vi "EditorEinfachCRIO-11-15.vi"() -> ()   [LabVIEW 2010]
panel:
  out "error out":errorcluster
  in  "MethodeLöschen":bool
  in  "Metavariablen":string[](array[string])
  in  "MethodeDuplizieren":bool
  out "Methoden":T1(array[cluster]) {"FPGAPID"."proportional gain (Kc)" format="%.11g"; "FPGAPID"."integral gain (Kc*Ts/Ti)" format="%.11g"; "FPGAPID"."derivative gain (Kc*Td/Ts)" format="%.11g"}
  in  "T_MainMach2":dbl[](array[numeric])
  in  "t_MainMach2":dbl[](array[numeric])
  in  "T_MainMach1":dbl[](array[numeric])
  in  "t_MainMach1":dbl[](array[numeric])
  in  "EinstellungenSpeichern":bool
  out "LangsameHeizungen":string[](array[string])
  in  "AllesSpeichern":bool
  in  "ModuleLH":i32[](array[numeric]) min=1 max=3 step=1
  in  "NamenLangsameHeizungen":string[](array[string])
  out "Schnelle Heizungen":string[](array[string])
  in  "Modul3/AIsNamen":string[](array[string])
  in  "Modul2/AIsNamen":string[](array[string])
  in  "Modul1/AIsNamen":string[](array[string])
  in  "Methodenname":string
  in  "Int.Stop2":dbl
  in  "Int.Start2":dbl
  in  "Int.Stop1":dbl
  in  "Int.Start1":dbl
  in  "ZeitpktMS-2":dbl
  in  "ZeitpktMS-1":dbl
  in  "SPMPV":i32[](array[numeric])
  in  "ZeitpunkteMPV":dbl[](array[numeric])
  in  "Regler für den Probenfluß":i32
  in  "DateinameECD2":string
  in  "DateiordnerECD2":path
  in  "DateinameECD1":string
  in  "DateiordnerECD1":path
  in  "Wert2":dbl
  in  "Vergleichsoperator2":dbl(ring) items=["<", "<=", "=", ">=", ">", "=/="]
  in  "AbfragbareVariablen2":dbl(ring) items=["T1-Trap1", "T1-Trap2", "T1-StirlingKühlkopf", "T1-PreCol1", "T1-PreCol2", "T1-MainCol1a", "T1-MainCol1b", "T1-MainCol2a", "T1-MainCol2b", "T1-Bronkhorst1a", "T1-Bronkhorst1b", "T1-Bronkhorst2a", "T1-Bronkhorst2b", "T1-2Pos1B", "T1-Spare9", "T1-2Pos1A", "T1-Spare10", "T1-TurboPump", "T1-StirlingPlatine", "T1-Spare5", "T1-Spare6", "T1-Spare7", "T1-Spare8", "F1-MFM1", "F1-MFM0D [mL]", "P1-MethaneHP", "P1-MethaneLP", "P1-Vacuum", "TurboSpeed", "I1-MS-AC", "I1-Trap1", "I1-Trap2", "T2-ECD1a", "T2-ECD1b", "T2-ECD2a", "T2-ECD2b", "T2-Col1a", "T2-Col1b", "T2-Col2a", "T2-Col2b", "T2-Spare1", "T2-Spare2", "T2-Oven_a", "T2-Oven_b", "T2-Spare3", "T2-Spare4", "T2-Spare5", "F2-MFM0", "F2-MFM2A", "F2-MFM2B", "P2-N2O_HP", "P2-N2O_LP", "P2-CO2_HP", "P2-CO2_LP", "AI-Spare1", "FL-MFM1000mL", "AI-Spare3", "AI-Spare4", "StirlingAlarm", "StirlingEmerg.", "AI-Spare7", "AI-Spare8", "AI-Spare9", "FL-MFM30mL", "T0-DC/DC5", "I0-24V_M0", "I0-48V_M1", "I0-24V_M1", "I0-28V_M2", "T0-Spare3", "T0-Spare2", "T0-Spare4", "T0-DC/DC7", "I0-20V_Laptop", "I0-28V_M1", "I0-24V_M2", "I0-12V_Licor", "T0-Spare1", "T0-Drier", "T0-Spare5", "F0-MFM0A [L]", "TL-Licor_a", "P0-Span-HP", "P0-spare1", "P0-Stickstoff-LP", "P0-Helium-LP", "P0-Cal-HP", "P0-P9Tavco[bar]", "F0-MFM0B [L]", "TL-Licor_b", "P0-Span-LP", "P0-spare2", "P0-Stickstoff-HP", "P0-Helium-HP", "P0-Cal-LP", "F0-MFM3", "T-Trap1", "T-Trap2", "T-PreMach1", "T-PreMach2", "T-MainMach1", "T-MainMach2", "PrC0", "PrC0-Licor", "PrC1-Säule2", "PrC1-Säule1", "MFC1-Sample", "MFC1-Methan", "PrC1-BackFlush1", "PrC1-BackFlush2", "MFC2A", "MFC2B", "MFC2C", "PrC2A", "MFC2D", "MFC2E", "PrC2B", "Gesamte Zeit", "Methodenzeit", "Zykluszeit Mod0", "Zykluszeit Mod1", "Zykluszeit Mod2A", "Zykluszeit Mod2B", "PositionMPV", "OverflowB", "OverflowA", "StirlingAlarmAlarm!"]
  in  "Dateiname Housekeeping":string
  in  "Dateiordner Housekeeping":path=path "C:/Users/Atmos/Desktop/Johnny"
  in  "Startmethode":i32=1
  in  "Dateien fürs MS schicken?":bool
  in  "Zwangsbedingungen":dbl[][](array[numeric])
  out "ZwangsBedingungen":string[][](array[string])
  in  "löschen":bool
  in  "Bedingung Nr. X":i32
  in  "Bedingung übernehmen":bool
  in  "Ausgangswert":dbl
  in  "BedienbareVariablen":dbl(ring) items=["D0-48V_M1", "D0-28V_M1", "D0-Pump2", "DL-LiCalS1H", "D-Spare2", "D-Spare4", "D0-28V_M2", "D0-Pump1", "D0-S01/EV1", "DL-Licor", "D0-EV3", "D0-EV2", "D1-StopMS", "D1-StartMS", "D1-TrapEvac1", "D1-TrapEvac2", "D1-2Pos1A", "D1-2Pos1B", "D1-TurboPump", "D1-PrePump", "D1-VacPump1", "D1-VacPump2", "D1-Stirling", "D1-P_MS", "D1-S1B(7)", "D1-S1A(6)", "D1-S1G", "D1-Fan3", "D1-LüfterMach1", "D1-LüfterMach2", "D1-MS-Power", "D2-SpülflußA", "D2-2Pos2B", "D2-2Pos2A", "D2-ECD1HeaterOff", "D2-Fan1", "D2-Fan2", "D2-Probe2A", "D2-Probe2B", "D2-SpülflußB", "D2-ECD2HeaterOff", "Servo1 an", "Servo2 an", "Servo1 kalt", "Servo2 kalt", "Heizen?Trap1", "Heizen?Trap2", "Heizen?PreMach1", "Heizen?PreMach2", "Heizen?MainMach1", "Heizen?MainMach2", "Methodennummer", "STOPP!!!", "H1-Valve1B heizen?", "H1-Bronkhorst1 heizen?", "H1-Bronkhorst2 heizen?", "H1-Valve1A heizen?", "H0-Drier heizen?", "HL-Licor heizen?", "H2-ECD2 heizen?", "H2-Oven heizen?", "H2-Spare1 heizen?", "H2-Col2 heizen?", "H2-Col1 heizen?", "H2-ECD1 heizen?", "PrC0", "PrC0-Licor", "PrC1-Säule2", "PrC1-Säule1", "MFC1-Sample", "MFC1-Methan", "PrC1-BackFlush1", "PrC1-BackFlush2", "MFC2A", "MFC2B", "MFC2C", "PrC2A", "MFC2D", "MFC2E", "PrC2B", "PositionMPV", "OverflowB", "OverflowA", "StirlingAlarmAlarm!"]
  in  "Wert1":dbl
  in  "Vergleichsoperator1":dbl(ring) items=["<", "<=", "=", ">=", ">", "=/="]
  in  "AbfragbareVariablen1":dbl(ring) items=["T1-Trap1", "T1-Trap2", "T1-StirlingKühlkopf", "T1-PreCol1", "T1-PreCol2", "T1-MainCol1a", "T1-MainCol1b", "T1-MainCol2a", "T1-MainCol2b", "T1-Bronkhorst1a", "T1-Bronkhorst1b", "T1-Bronkhorst2a", "T1-Bronkhorst2b", "T1-2Pos1B", "T1-Spare9", "T1-2Pos1A", "T1-Spare10", "T1-TurboPump", "T1-StirlingPlatine", "T1-Spare5", "T1-Spare6", "T1-Spare7", "T1-Spare8", "F1-MFM1", "F1-MFM0D [mL]", "P1-MethaneHP", "P1-MethaneLP", "P1-Vacuum", "TurboSpeed", "I1-MS-AC", "I1-Trap1", "I1-Trap2", "T2-ECD1a", "T2-ECD1b", "T2-ECD2a", "T2-ECD2b", "T2-Col1a", "T2-Col1b", "T2-Col2a", "T2-Col2b", "T2-Spare1", "T2-Spare2", "T2-Oven_a", "T2-Oven_b", "T2-Spare3", "T2-Spare4", "T2-Spare5", "F2-MFM0", "F2-MFM2A", "F2-MFM2B", "P2-N2O_HP", "P2-N2O_LP", "P2-CO2_HP", "P2-CO2_LP", "AI-Spare1", "FL-MFM1000mL", "AI-Spare3", "AI-Spare4", "StirlingAlarm", "StirlingEmerg.", "AI-Spare7", "AI-Spare8", "AI-Spare9", "FL-MFM30mL", "T0-DC/DC5", "I0-24V_M0", "I0-48V_M1", "I0-24V_M1", "I0-28V_M2", "T0-Spare3", "T0-Spare2", "T0-Spare4", "T0-DC/DC7", "I0-20V_Laptop", "I0-28V_M1", "I0-24V_M2", "I0-12V_Licor", "T0-Spare1", "T0-Drier", "T0-Spare5", "F0-MFM0A [L]", "TL-Licor_a", "P0-Span-HP", "P0-spare1", "P0-Stickstoff-LP", "P0-Helium-LP", "P0-Cal-HP", "P0-P9Tavco[bar]", "F0-MFM0B [L]", "TL-Licor_b", "P0-Span-LP", "P0-spare2", "P0-Stickstoff-HP", "P0-Helium-HP", "P0-Cal-LP", "F0-MFM3", "T-Trap1", "T-Trap2", "T-PreMach1", "T-PreMach2", "T-MainMach1", "T-MainMach2", "PrC0", "PrC0-Licor", "PrC1-Säule2", "PrC1-Säule1", "MFC1-Sample", "MFC1-Methan", "PrC1-BackFlush1", "PrC1-BackFlush2", "MFC2A", "MFC2B", "MFC2C", "PrC2A", "MFC2D", "MFC2E", "PrC2B", "Gesamte Zeit", "Methodenzeit", "Zykluszeit Mod0", "Zykluszeit Mod1", "Zykluszeit Mod2A", "Zykluszeit Mod2B", "PositionMPV", "OverflowB", "OverflowA", "StirlingAlarmAlarm!"]
  in  "AIsNamenZurücksetzen":bool
  in  "Methode Nummer":i32
  in  "MethodeLaden":bool
  in  "EditorBeenden":bool
  out "AnzahlRegler/Modul":i32[](array[numeric])
  in  "PIDs für \"träge\" Heizungen":T2(array[cluster])
  in  "AIsLH":i32[](array[numeric]) min=0 max=31 step=1
  in  "Traps/MachsKoeff":dbl[][](array[numeric])=[[0.0, 0.0, 0.0, 0.0, 0.0, 0.0, 0.0, 0.0, 0.0, 0.0, 0.0, 0.0, 0.0, 0.0, 0.0, 0.0, 0.0, 0.0, 0.0, 0.0, 0.0, 0.0, 0.0, 0.0, 0.0, 0.0, 0.0, 0.0, 0.0, 0.0, 0.0, 0.0]]
  in  "Modul3/AI koeff":dbl[][](array[numeric])=[[0.0, 0.0, 0.0, 0.0, 0.0, 0.0, 0.0, 0.0, 0.0, 0.0, 0.0, 0.0, 0.0, 0.0, 0.0, 0.0, 0.0, 0.0, 0.0, 0.0, 0.0, 0.0, 0.0, 0.0, 0.0, 0.0, 0.0, 0.0, 0.0, 0.0, 0.0, 0.0]]
  in  "Modul2/AI koeff":dbl[][](array[numeric])=[[0.0, 0.0, 0.0, 0.0, 0.0, 0.0, 0.0, 0.0, 0.0, 0.0, 0.0, 0.0, 0.0, 0.0, 0.0, 0.0, 0.0, 0.0, 0.0, 0.0, 0.0, 0.0, 0.0, 0.0, 0.0, 0.0, 0.0, 0.0, 0.0, 0.0, 0.0, 0.0]]
  in  "Modul1/AI koeff":dbl[][](array[numeric])=[[0.0, 0.0, 0.0, 0.0, 0.0, 0.0, 0.0, 0.0, 0.0, 0.0, 0.0, 0.0, 0.0, 0.0, 0.0, 0.0, 0.0, 0.0, 0.0, 0.0, 0.0, 0.0, 0.0, 0.0, 0.0, 0.0, 0.0, 0.0, 0.0, 0.0, 0.0, 0.0]]
  in  "T_PreMach2":dbl[](array[numeric])
  in  "t_PreMach2":dbl[](array[numeric])
  in  "T_PreMach1":dbl[](array[numeric])
  in  "t_PreMach1":dbl[](array[numeric])
  in  "SHSetpoints":dbl[][](array[numeric])
  in  "ZeitpktFPGAFixp":dbl[](array[numeric])
  in  "FPGAPID":T3(array[cluster]) {"proportional gain (Kc)" format="%.11g"; "integral gain (Kc*Ts/Ti)" format="%.11g"; "derivative gain (Kc*Td/Ts)" format="%.11g"}
  in  "ZeitpktFPGAPID":dbl[](array[numeric])
  in  "FPGABoolesch":bool[][](array[boolean])
  in  "ZPktFPGABoolesch":dbl[](array[numeric])
  in  "LHHeizen?":bool[](array[boolean])
  in  "LHSetpoints":dbl[](array[numeric])
  out "HorstMod1Name":string[](array[string])
  out "HorstMod2AName":string[](array[string])
  out "HorstMod2BName":string[](array[string])
  in  "HorstSPMod1":dbl[][](array[numeric])
  in  "HorstSPMod2A":dbl[][](array[numeric])
  in  "HorstSPMod2B":dbl[][](array[numeric])
  in  "Mod1HorstZeitpkt":dbl[](array[numeric])
  in  "Mod2AHorstZeitpkt":dbl[](array[numeric])
  in  "Mod2BHorstZeitpkt":dbl[](array[numeric])
  in  "HorstSPMod0":dbl[][](array[numeric])
  out "HorstMod0Name":string[](array[string])
  in  "Mod0HorstZeitpkt":dbl[](array[numeric])
  in  "MWAntwortMod2B":string[](array[string])=[":060F020121", ":0610020121", ":0611020121"]
  in  "MWAntwortMod2A":string[](array[string])=[":060F020121", ":0610020121", ":0611020121"]
  in  "MWAntwortMod1":string[](array[string])=[":060F020121", ":0610020121", ":0611020121"]
  in  "MWAntwortMod0":string[](array[string])=[":060F020121", ":0610020121", ":0611020121"]
  in  "FaktorMod2B":dbl[](array[numeric])=[9.375e-05, 9.375e-05, 9.375e-05]
  in  "FaktorMod2A":dbl[](array[numeric])=[9.375e-05, 9.375e-05, 9.375e-05]
  in  "FaktorMod1":dbl[](array[numeric])=[9.375e-05, 9.375e-05, 9.375e-05]
  in  "FaktorMod0":dbl[](array[numeric])=[9.375e-05, 9.375e-05, 9.375e-05]
  in  "SPvorgebenMod2B":string[](array[string])=[":060F020121", ":0610020121", ":0611020121"]
  in  "SPvorgebenMod2A":string[](array[string])=[":060F020121", ":0610020121", ":0611020121"]
  in  "SPvorgebenMod1":string[](array[string])=[":060F020121", ":0610020121", ":0611020121"]
  in  "SPvorgebenMod0":string[](array[string])=[":060F020121", ":0610020121", ":0611020121"]
  in  "MWabfragenMod2B":string[](array[string])=[":060F0401210120", ":06100401210120", ":06110401210120"]
  in  "MWabfragenMod2A":string[](array[string])=[":060F0401210120", ":06100401210120", ":06110401210120"]
  in  "MWabfragenMod1":string[](array[string])=[":060F0401210120", ":06100401210120", ":06110401210120"]
  in  "MWabfragenMod0":string[](array[string])=[":060F0401210120", ":06100401210120", ":06110401210120"]
  in  "ReglerNameMod2B":string[](array[string])
  in  "ReglerNameMod2A":string[](array[string])
  in  "ReglerNameMod1":string[](array[string])
  in  "ReglerNameMod0":string[](array[string])
  in  "DIOsSPMod2B":bool[][](array[boolean])
  in  "DIOsSPMod2A":bool[][](array[boolean])
  in  "DIOsSPMod1":bool[][](array[boolean])
  in  "ZeitpktDIOsMod2B":dbl[](array[numeric])
  in  "ZeitpktDIOsMod2A":dbl[](array[numeric])
  in  "ZeitpktDIOsMod1":dbl[](array[numeric])
  out "DIOsMod2BName":string[](array[string])
  out "DIOsMod2AName":string[](array[string])
  out "DIOsMod1Name":string[](array[string])
  out "DIOsMod0Name":string[](array[string])
  in  "DIOsSPMod0":bool[][](array[boolean])
  in  "ZeitpktDIOsMod0":dbl[](array[numeric])
  in  "MethodeSpeichern":bool
  in  "EinstellungenFertig":bool
  in  "DIOsMod2BName":string[](array[string])
  in  "DIOsMod2AName":string[](array[string])
  in  "DIOsMod1Name":string[](array[string])
  in  "DIOsMod0Name":string[](array[string])
  in  "Zykluslängen [s]":dbl[](array[numeric])
  in  "DIOsMod2BNr":i32[](array[numeric]) min=0 max=63 step=1
  in  "DIOsMod2ANr":i32[](array[numeric]) min=0 max=63 step=1
  in  "DIOsMod1Nr":i32[](array[numeric]) min=0 max=63 step=1
  in  "DIOsMod0Nr":i32[](array[numeric]) min=0 max=63 step=1
  # "Hier gehts lang!"
  # "Hier gehts lang!"
  # "Servo1         Servo2        Servo1        Servo2          Trap1          Trap2      PreMach1  PreMach2 MainMach1 MainMach2\n        an                 an              kalt             kalt            heizen         heizen        heizen         heizen         heizen         heizen"
  # "Trap1"
  # "Trap2"
  # "PreMach1"
  # "PreMach2"
  # "MainMach1"
  # "MainMach2"
  # "Die Analogeingänge sind entsprechend der AI-Module des CRIO angeordnet (3x32); es wird eine quadratische Kennlinie angenommen, also: y=a0+a1*x+a2*x^2;\ndie drei Koeffizienten werden in dieser Reihenfolge eingegeben (v.l.n.r.): a0, a1, a2."
  # "Vorsicht!!! Wer hier nicht ganz genau weiß, was er tut, läßt bitte die Finger davon!\nDie Heizungen werden über den FPGA gesteuert, d.h. wenn man die Anzahl oder \ndie Anschlüsse der Heizungen ändert, muß das FPGA-Programm entsprechend\nangepaßt werden.\nModuleLH bezieht sich auf die drei AI-Module des CRIO (1,2,3) und AIsLH auf den\nAnschluß im jeweiligen Modul."
  # "Die digitalen Ein-/Ausgänge werden modulweise aufgelistet (0, 1, 2A, 2B) und benannt; die zugehörigen Anschlüsse\nwerden folgendermaßen durchgezählt: DIO 0...31 von Modul5 entspricht hier 0...31; DIO 0...31 von Modul6 entspricht hier 32+(0...31)=32...63."
  # "Im weiteren können beliebig viele Methoden definiert werden; mit welcher davon soll das Programm starten? Die erste Methode trägt die Nummer 0."
  # "Sososo... alle Einstellungen vorgenommen? Wirklich alle? Sicher? Bereit, mit den Methoden fortzufahren? Na super, dann trau Dich und drück den Knopf!"
  # "Es können beliebig viele Methoden definiert werden; die gewünschte Nummer auswählen und die entsprechende Methode laden, dann nach Belieben dran rumfummeln und anschließend, wenns beliebt, die vorgenommenen Änderungen an der Methode übernehmen (das bedeutet NICHT, daß die Änderungen in einer Datei abgelegt werden, dafür gibts nen extra Knopp);\n\"Editor beenden\" dürfte klar sein. Und Tschüß!"
  # ":::Tom \"Awesome\"  Burner Jr.:::"
  # "Sollen die Daten vom MS abgefragt werden? Wenn ja, zu welchen Zeitpunkten (im Zyklus1)?"
  # "Schnelle Heizungen..."
  # "Die eingegebenen Punkte im (t-T)-Raum werden durch lineare Funktionen verbunden, jeweils definiert von Punkt zu Punkt."
  # "Stellung des Multipositionsventils; die Zeitpunkte beziehen sich auf den Zyklus von Modul0.\nDie Stellungen bezeichnen: \n1. Cal - 2. Span - 3. ? - 4. ? - \n5. Plank - 6. Air - 7. ?"
  # "Innerhalb welcher Zeitfenster (Modul1) soll der Probenfluß integriert werden?"
  # "Der Gipfel der Flexibilität: die Zwangsbedingungen!\nBitte boolesche Werte als 0/1 eingeben"
  # "Dran denken: die Daten werden auf dem CRIO\nabgelegt, nicht auf dem Notebook;\nDateinamen bitte ohne Pfad und .tdms eingeben"
  # "Die Bronkhorst-Regler werden modulweise zusammengefasst an den CRIO \nangeschlossen, Mod0 an Port0, Mod1 an Port1, Mod2A&2B an Port2;\ndie Strings für die Steuerung und Abfrage der Regler ergeben sich aus dem bronkhorstschen Handbuch; der Faktor berechnet sich durch \"Vollausschlag des Reglers (in der gewünschten Einheit, z.B. Bar)\"/32000;\n'Regler für den Probenfluß' meint die Nummer des entsprechenden Reglers in der Liste aller Regler, wobei der erste die Nummer 0 trägt."
  # "Mod0\n\nMod1\n\nMod2A\n\nMod2B"
  # "UND"
  # "TSetpTrap1               TMaxTrap1              TSetpTrap2              TMaxTrap2             TMaxPreMach1      TMaxPreMach2        TMaxMainMach1      TMaxMainMach2"
  # "Wer will noch mehr, wer hat noch nichts? An dieser Stelle können weitere Variablen definiert werden, mit deren Hilfe die Zwangsbedingungen erst ihre volle Pracht und Mächtigkeit entfalten. Alle Variablen sind numerische Größen und haben damit beliebig viele Zustände. Beim Programmstart werden sie mit Null initialisiert.\nHöchschte Vorsicht ist beim Umbenennen oder gar Löschen von Variablen geboten, weil sich das fatal auf bestehende Zwangsbedingungen auswirken kann. Am besten immer nur neue Variablen hinzufügen, das garantiert sicheren Spaß ohne Spätfolgen."
types:
  T1 = cluster{"Zykluslängen [s]":dbl[], "ZeitpktDIOsMod0":dbl[], "ZeitpktDIOsMod1":dbl[], "ZeitpktDIOsMod2A":dbl[], "ZeitpktDIOsMod2B":dbl[], "DIOsSPMod0":bool[][], "DIOsSPMod1":bool[][], "DIOsSPMod2A":bool[][], "DIOsSPMod2B":bool[][], "Mod0HorstZeitpkt":dbl[], "Mod1HorstZeitpkt":dbl[], "Mod2AHorstZeitpkt":dbl[], "Mod2BHorstZeitpkt":dbl[], "HorstSPMod0":dbl[][], "HorstSPMod1":dbl[][], "HorstSPMod2A":dbl[][], "HorstSPMod2B":dbl[][], "LHSetpoints":dbl[], "LHHeizen?":bool[], "ZPktFPGABoolesch":dbl[], "FPGABoolesch":bool[][], "ZeitpktFPGAPID":dbl[], "FPGAPID":cluster{"proportional gain (Kc)":fxp<+/-,16,8>, "integral gain (Kc*Ts/Ti)":fxp<+/-,16,8>, "derivative gain (Kc*Td/Ts)":fxp<+/-,16,8>}[][], "ZeitpktFPGAFixp":dbl[], "SHSetpoints":dbl[][], "t_PreMach1":dbl[], "T_PreMach1":dbl[], "t_PreMach2":dbl[], "T_PreMach2":dbl[], "PIDs für \"träge\" Heizungen":cluster{"proportional gain (Kc)":dbl, "integral time (Ti, min)":dbl, "derivative time (Td, min)":dbl}[], "Zwangsbedingungen":dbl[][], "Dateien fürs MS schicken?":bool, "ZeitpunkteMPV":dbl[], "SPMPV":i32[], "ZeitpktMS-1":dbl, "ZeitpktMS-2":dbl, "Int.Start1":dbl, "Int.Stop1":dbl, "Int.Start2":dbl, "Int.Stop2":dbl, "Methodenname":string, "t_MainMach1":dbl[], "T_MainMach1":dbl[], "t_MainMach2":dbl[], "T_MainMach2":dbl[]}[]
  T2 = cluster{"proportional gain (Kc)":dbl, "integral time (Ti, min)":dbl, "derivative time (Td, min)":dbl}[]
  T3 = cluster{"proportional gain (Kc)":fxp<+/-,16,8>, "integral gain (Kc*Ts/Ti)":fxp<+/-,16,8>, "derivative gain (Kc*Td/Ts)":fxp<+/-,16,8>}[][]
  T4 = cluster{"DIOsMod0Nr":i32[], "DIOsMod1Nr":i32[], "DIOsMod2ANr":i32[], "DIOsMod2BNr":i32[], "AIsLH":i32[], "AnzahlRegler/Modul":i32[], "Regler für den Probenfluß":i32, "SPvorgebenMod0":string[], "SPvorgebenMod1":string[], "SPvorgebenMod2A":string[], "SPvorgebenMod2B":string[], "MWAntwortMod0":string[], "MWAntwortMod1":string[], "MWAntwortMod2A":string[], "MWAntwortMod2B":string[], "FaktorMod0":dbl[], "FaktorMod1":dbl[], "FaktorMod2A":dbl[], "FaktorMod2B":dbl[], "MWabfragenMod0":string[], "MWabfragenMod1":string[], "MWabfragenMod2A":string[], "MWabfragenMod2B":string[], "Modul1/AI koeff":dbl[][], "Modul2/AI koeff":dbl[][], "Modul3/AI koeff":dbl[][], "Traps/MachsKoeff":dbl[][], "Modul1/AIsNamen":string[], "Modul2/AIsNamen":string[], "Modul3/AIsNamen":string[], "DIOsMod0Name":string[], "DIOsMod1Name":string[], "DIOsMod2AName":string[], "DIOsMod2BName":string[], "ReglerNameMod0":string[], "ReglerNameMod1":string[], "ReglerNameMod2A":string[], "ReglerNameMod2B":string[], "Startmethode":i32, "Dateiordner Housekeeping":path, "Dateiname Housekeeping":string, "DateiordnerECD1":path, "DateinameECD1":string, "DateiordnerECD2":path, "DateinameECD2":string, "NamenLangsameHeizungen":string[], "ModuleLH":i32[], "Metavariablen":string[]}
  T5 = enum16{"open", "replace", "create", "open or create", "replace or create", "replace or create with confirmation"}
  T6 = cluster{"Zykluslängen [s]":dbl[], "ZeitpktDIOsMod0":dbl[], "ZeitpktDIOsMod1":dbl[], "ZeitpktDIOsMod2A":dbl[], "ZeitpktDIOsMod2B":dbl[], "DIOsSPMod0":bool[][], "DIOsSPMod1":bool[][], "DIOsSPMod2A":bool[][], "DIOsSPMod2B":bool[][], "Mod0HorstZeitpkt":dbl[], "Mod1HorstZeitpkt":dbl[], "Mod2AHorstZeitpkt":dbl[], "Mod2BHorstZeitpkt":dbl[], "HorstSPMod0":dbl[][], "HorstSPMod1":dbl[][], "HorstSPMod2A":dbl[][], "HorstSPMod2B":dbl[][], "LHSetpoints":dbl[], "LHHeizen?":bool[], "ZPktFPGABoolesch":dbl[], "FPGABoolesch":bool[][], "ZeitpktFPGAPID":dbl[], "FPGAPID":cluster{"proportional gain (Kc)":fxp<+/-,16,8>, "integral gain (Kc*Ts/Ti)":fxp<+/-,16,8>, "derivative gain (Kc*Td/Ts)":fxp<+/-,16,8>}[][], "ZeitpktFPGAFixp":dbl[], "SHSetpoints":dbl[][], "t_PreMach1":dbl[], "T_PreMach1":dbl[], "t_PreMach2":dbl[], "T_PreMach2":dbl[], "PIDs für \"träge\" Heizungen":cluster{"proportional gain (Kc)":dbl, "integral time (Ti, min)":dbl, "derivative time (Td, min)":dbl}[], "Zwangsbedingungen":dbl[][], "Dateien fürs MS schicken?":bool, "ZeitpunkteMPV":dbl[], "SPMPV":i32[], "ZeitpktMS-1":dbl, "ZeitpktMS-2":dbl, "Int.Start1":dbl, "Int.Stop1":dbl, "Int.Start2":dbl, "Int.Stop2":dbl, "Methodenname":string, "t_MainMach1":dbl[], "T_MainMach1":dbl[], "t_MainMach2":dbl[], "T_MainMach2":dbl[]}
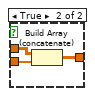
[diagram p9: hidden frame]
diagram:
  n1 = Open/Create/Replace File(file path (use dialog)=path "c:/einstellungen.per" ("Dateipfad Einstellungen")) -> (refnum out=w20:refnum<file>, error out=w21:errorcluster)  [unwired: 5 in, 1 out]
  n2 = Read from Binary File(5:T4 {"DIOsMod0Nr"=[], "DIOsMod1Nr"=[], "DIOsMod2ANr"=[], "DIOsMod2BNr"=[], "AIsLH"=[], "AnzahlRegler/Modul"=[], "Regler für den Probenfluß"=0, "SPvorgebenMod0"=[], "SPvorgebenMod1"=[], "SPvorgebenMod2A"=[], "SPvorgebenMod2B"=[], "MWAntwortMod0"=[], "MWAntwortMod1"=[], "MWAntwortMod2A"=[], "MWAntwortMod2B"=[], "FaktorMod0"=[], "FaktorMod1"=[], "FaktorMod2A"=[], "FaktorMod2B"=[], "MWabfragenMod0"=[], "MWabfragenMod1"=[], "MWabfragenMod2A"=[], "MWabfragenMod2B"=[], "Modul1/AI koeff"=[], "Modul2/AI koeff"=[], "Modul3/AI koeff"=[], "Traps/MachsKoeff"=[], "Modul1/AIsNamen"=[], "Modul2/AIsNamen"=[], "Modul3/AIsNamen"=[], "DIOsMod0Name"=[], "DIOsMod1Name"=[], "DIOsMod2AName"=[], "DIOsMod2BName"=[], "ReglerNameMod0"=[], "ReglerNameMod1"=[], "ReglerNameMod2A"=[], "ReglerNameMod2B"=[], "Startmethode"=0, "Dateiordner Housekeeping"=path "", "Dateiname Housekeeping"="", "DateiordnerECD1"=path "", "DateinameECD1"="", "DateiordnerECD2"=path "", "DateinameECD2"="", "NamenLangsameHeizungen"=[], "ModuleLH"=[], "Metavariablen"=[]} ("Ausgangs-Cluster"), 8:w21, 11:w20) -> (0:w18:errorcluster, 2:w1:T4, 3:w19:refnum<file>)  [unwired: 3 in, 1 out]
  n3 = flat-sequence {
    tunnel: w1 -> [w87]
    tunnel: [w40] -> w7
    tunnel: [w110] -> w37
    tunnel: [w109] -> w36
    tunnel: [w108] -> w35
    tunnel: [w107] -> w34
    tunnel: [w106] -> w33
    tunnel: [w105] -> w32
    tunnel: [w104] -> w31
    tunnel: [w103] -> w30
    tunnel: [w102] -> w29
    tunnel: [w97] -> w28
    tunnel: [w96] -> w27
    tunnel: [w95] -> w26
    tunnel: [w94] -> w25
    tunnel: [w93] -> w24
    tunnel: [w92] -> w23
    tunnel: w16 -> [w91]
    tunnel: [w90] -> w8
    tunnel: w7 -> [w90]
    tunnel: [w89] -> w4
    tunnel: [w88] -> w3
    tunnel: w37 -> [w219]
    tunnel: w36 -> [w218]
    tunnel: w35 -> [w217]
    tunnel: w34 -> [w216]
    tunnel: w33 -> [w215]
    tunnel: w32 -> [w214]
    tunnel: w31 -> [w212]
    tunnel: w30 -> [w213]
    tunnel: w29 -> [w211]
    tunnel: w28 -> [w195]
    tunnel: w27 -> [w209]
    tunnel: w26 -> [w208]
    tunnel: w25 -> [w207]
    tunnel: w24 -> [w206]
    tunnel: w6 -> [w205]
    tunnel: w23 -> [w199]
    tunnel: w9 -> [w198]
    tunnel: w8 -> [w194]
    tunnel: w4 -> [w192]
    tunnel: w3 -> [w190]
    frame #0 {
      n4 = Unbundle(w87) -> ("DIOsMod0Nr"=w86:i32[], "DIOsMod1Nr"=w85:i32[], "DIOsMod2ANr"=w84:i32[], "DIOsMod2BNr"=w83:i32[], "AIsLH"=w82:i32[], "AnzahlRegler/Modul"=w81:i32[], "Regler für den Probenfluß"=w80:i32, "SPvorgebenMod0"=w79:string[], "SPvorgebenMod1"=w78:string[], "SPvorgebenMod2A"=w77:string[], "SPvorgebenMod2B"=w76:string[], "MWAntwortMod0"=w75:string[], "MWAntwortMod1"=w74:string[], "MWAntwortMod2A"=w73:string[], "MWAntwortMod2B"=w72:string[], "FaktorMod0"=w71:dbl[], "FaktorMod1"=w70:dbl[], "FaktorMod2A"=w69:dbl[], "FaktorMod2B"=w68:dbl[], "MWabfragenMod0"=w67:string[], "MWabfragenMod1"=w66:string[], "MWabfragenMod2A"=w65:string[], "MWabfragenMod2B"=w64:string[], "Modul1/AI koeff"=w63:dbl[][], "Modul2/AI koeff"=w62:dbl[][], "Modul3/AI koeff"=w61:dbl[][], "Traps/MachsKoeff"=w60:dbl[][], "Modul1/AIsNamen"=w59:string[], "Modul2/AIsNamen"=w58:string[], "Modul3/AIsNamen"=w57:string[], "DIOsMod0Name"=w56:string[], "DIOsMod1Name"=w55:string[], "DIOsMod2AName"=w54:string[], "DIOsMod2BName"=w53:string[], "ReglerNameMod0"=w52:string[], "ReglerNameMod1"=w51:string[], "ReglerNameMod2A"=w50:string[], "ReglerNameMod2B"=w49:string[], "Startmethode"=w48:i32, "Dateiordner Housekeeping"=w38:path, "Dateiname Housekeeping"=w47:string, "DateiordnerECD1"=w46:path, "DateinameECD1"=w45:string, "DateiordnerECD2"=w44:path, "DateinameECD2"=w43:string, "NamenLangsameHeizungen"=w40:string[], "ModuleLH"=w41:i32[], "Metavariablen"=w39:string[])
      n5 = invoke on="MethodeLöschen" class="Bool (strict)" method="Reinit To Default"() -> ()  [unwired: 3 in, 3 out]
      n6 = property on="ModuleLH" class="Arr (strict)"("Value"=w41) -> ()  [unwired: 2 in, 2 out]
      n7 = property on="AIsLH" class="Arr (strict)"("Value"=w82) -> ()  [unwired: 2 in, 2 out]
      n8 = property on="Dateiname Housekeeping" class="Str"("Value"=w47) -> ()  [unwired: 2 in, 2 out]
      n9 = property on="DIOsMod0Nr" class="Arr (strict)"("Value"=w86) -> ()  [unwired: 2 in, 2 out]
      n10 = property on="DateiordnerECD1" class="Path"("Value"=w46) -> ()  [unwired: 2 in, 2 out]
      n11 = property on="DIOsMod1Nr" class="Arr (strict)"("Value"=w85) -> ()  [unwired: 2 in, 2 out]
      n12 = property on="DateinameECD1" class="Str"("Value"=w45) -> ()  [unwired: 2 in, 2 out]
      n13 = property on="DateiordnerECD2" class="Path"("Value"=w44) -> ()  [unwired: 2 in, 2 out]
      n14 = property on="DateinameECD2" class="Str"("Value"=w43) -> ()  [unwired: 2 in, 2 out]
      n15 = property on="DIOsMod2ANr" class="Arr (strict)"("Value"=w84) -> ()  [unwired: 2 in, 2 out]
      n16 = property on="NamenLangsameHeizungen" class="Arr (strict)"("Value"=w40) -> ()  [unwired: 2 in, 2 out]
      n17 = property on="Metavariablen" class="Arr (strict)"("Value"=w39) -> ()  [unwired: 2 in, 2 out]
      n18 = property on="DIOsMod2BNr" class="Arr (strict)"("Value"=w83) -> ()  [unwired: 2 in, 2 out]
      n19 = property on="AnzahlRegler/Modul" class="Arr (strict)"("Value"=w81) -> ()  [unwired: 2 in, 2 out]
      n20 = property on="Regler für den Probenfluß" class="DigNum (strict)"("Value"=w80) -> ()  [unwired: 2 in, 2 out]
      n21 = property on="SPvorgebenMod0" class="Arr (strict)"("Value"=w79) -> ()  [unwired: 2 in, 2 out]
      n22 = property on="ReglerNameMod2B" class="Arr (strict)"("Value"=w49) -> ()  [unwired: 2 in, 2 out]
      n23 = property on="Startmethode" class="DigNum (strict)"("Value"=w48) -> ()  [unwired: 2 in, 2 out]
      n24 = property on="Dateiordner Housekeeping" class="Path"("Value"=w38) -> ()  [unwired: 2 in, 2 out]
      n25 = property on="SPvorgebenMod1" class="Arr (strict)"("Value"=w78) -> ()  [unwired: 2 in, 2 out]
      n26 = property on="SPvorgebenMod2A" class="Arr (strict)"("Value"=w77) -> ()  [unwired: 2 in, 2 out]
      n27 = property on="SPvorgebenMod2B" class="Arr (strict)"("Value"=w76) -> ()  [unwired: 2 in, 2 out]
      n28 = property on="MWAntwortMod0" class="Arr (strict)"("Value"=w75) -> ()  [unwired: 2 in, 2 out]
      n29 = property on="MWAntwortMod1" class="Arr (strict)"("Value"=w74) -> ()  [unwired: 2 in, 2 out]
      n30 = property on="MWAntwortMod2A" class="Arr (strict)"("Value"=w73) -> ()  [unwired: 2 in, 2 out]
      n31 = property on="MWAntwortMod2B" class="Arr (strict)"("Value"=w72) -> ()  [unwired: 2 in, 2 out]
      n32 = property on="FaktorMod0" class="Arr (strict)"("Value"=w71) -> ()  [unwired: 2 in, 2 out]
      n33 = property on="FaktorMod1" class="Arr (strict)"("Value"=w70) -> ()  [unwired: 2 in, 2 out]
      n34 = property on="FaktorMod2B" class="Arr (strict)"("Value"=w68) -> ()  [unwired: 2 in, 2 out]
      n35 = property on="MWabfragenMod0" class="Arr (strict)"("Value"=w67) -> ()  [unwired: 2 in, 2 out]
      n36 = property on="FaktorMod2A" class="Arr (strict)"("Value"=w69) -> ()  [unwired: 2 in, 2 out]
      n37 = property on="MWabfragenMod1" class="Arr (strict)"("Value"=w66) -> ()  [unwired: 2 in, 2 out]
      n38 = property on="MWabfragenMod2A" class="Arr (strict)"("Value"=w65) -> ()  [unwired: 2 in, 2 out]
      n39 = property on="MWabfragenMod2B" class="Arr (strict)"("Value"=w64) -> ()  [unwired: 2 in, 2 out]
      n40 = property on="Modul1/AI koeff" class="Arr (strict)"("Value"=w63) -> ()  [unwired: 2 in, 2 out]
      n41 = property on="Modul3/AI koeff" class="Arr (strict)"("Value"=w61) -> ()  [unwired: 2 in, 2 out]
      n42 = property on="Traps/MachsKoeff" class="Arr (strict)"("Value"=w60) -> ()  [unwired: 2 in, 2 out]
      n43 = property on="Modul1/AIsNamen" class="Arr (strict)"("Value"=w59) -> ()  [unwired: 2 in, 2 out]
      n44 = property on="Modul2/AIsNamen" class="Arr (strict)"("Value"=w58) -> ()  [unwired: 2 in, 2 out]
      n45 = property on="Modul3/AIsNamen" class="Arr (strict)"("Value"=w57) -> ()  [unwired: 2 in, 2 out]
      n46 = property on="Modul2/AI koeff" class="Arr (strict)"("Value"=w62) -> ()  [unwired: 2 in, 2 out]
      n47 = property on="DIOsMod0Name" class="Arr (strict)"("Value"=w56) -> ()  [unwired: 2 in, 2 out]
      n48 = property on="DIOsMod1Name" class="Arr (strict)"("Value"=w55) -> ()  [unwired: 2 in, 2 out]
      n49 = property on="DIOsMod2AName" class="Arr (strict)"("Value"=w54) -> ()  [unwired: 2 in, 2 out]
      n50 = property on="DIOsMod2BName" class="Arr (strict)"("Value"=w53) -> ()  [unwired: 2 in, 2 out]
      n51 = property on="ReglerNameMod0" class="Arr (strict)"("Value"=w52) -> ()  [unwired: 2 in, 2 out]
      n52 = property on="ReglerNameMod1" class="Arr (strict)"("Value"=w51) -> ()  [unwired: 2 in, 2 out]
      n53 = property on="ReglerNameMod2A" class="Arr (strict)"("Value"=w50) -> ()  [unwired: 2 in, 2 out]
      "Schnelle Heizungen" <- string[] ["U[V]Trap1", "U[V]Trap2", "U[V]PreMach1", "U[V]PreMach2", "U[V]MainMach1", "U[V]MainMach2"]
    }
    frame #1 {
      n54 = while {
        tunnel: ["DIOsMod0Name"] -> w110
        tunnel: ["DIOsMod1Name"] -> w109
        tunnel: ["DIOsMod2AName"] -> w108
        tunnel: ["DIOsMod2BName"] -> w107
        tunnel: ["ReglerNameMod0"] -> w106
        tunnel: ["ReglerNameMod1"] -> w105
        tunnel: ["ReglerNameMod2A"] -> w104
        tunnel: ["ReglerNameMod2B"] -> w103
        tunnel: [w119] -> w102
        tunnel: ["ReglerNameMod2B"] -> w101
        tunnel: ["ReglerNameMod2A"] -> w100
        tunnel: ["ReglerNameMod1"] -> w99
        tunnel: ["ReglerNameMod0"] -> w98
        tunnel: ["DIOsMod0Name"] -> w96
        tunnel: ["DIOsMod1Name"] -> w95
        tunnel: ["DIOsMod2AName"] -> w94
        tunnel: ["DIOsMod2BName"] -> w93
        tunnel: ["NamenLangsameHeizungen"] -> w92
        tunnel: w91 -> [w114]
        tunnel: ["Metavariablen"] -> w89
        tunnel: ["Metavariablen"] -> w88
        stop <- "EinstellungenFertig" stop-if-true
        n55 = Wait (ms)(milliseconds to wait=u32 500 ("Zu wartende ms")) -> ()  [unwired: 1 out]
        n56 = case shown="True" "AIsNamenZurücksetzen" {
          frame False {
          }
          frame True {
            w185 = 32 ("Länge")
            w186 = string[] ["Mod1/AI0", "Mod1/AI1", "Mod1/AI2", "Mod1/AI3", "Mod1/AI4", "Mod1/AI5", "Mod1/AI6", "Mod1/AI7", "Mod1/AI8", "Mod1/AI9", "Mod1/AI10", "Mod1/AI11", "Mod1/AI12", "Mod1/AI13", "Mod1/AI14", "Mod1/AI15", "Mod1/AI16", "Mod1/AI17", "Mod1/AI18", "Mod1/AI19", "Mod1/AI20", "Mod1/AI21", "Mod1/AI22", "Mod1/AI23", "Mod1/AI24", "Mod1/AI25", "Mod1/AI26", "Mod1/AI27", "Mod1/AI28", "Mod1/AI29", "Mod1/AI30", "Mod1/AI31", "Mod2/AI0", "Mod2/AI1", "Mod2/AI2", "Mod2/AI3", "Mod2/AI4", "Mod2/AI5", "Mod2/AI6", "Mod2/AI7", "Mod2/AI8", "Mod2/AI9", "Mod2/AI10", "Mod2/AI11", "Mod2/AI12", "Mod2/AI13", "Mod2/AI14", "Mod2/AI15", "Mod2/AI16", "Mod2/AI17", "Mod2/AI18", "Mod2/AI19", "Mod2/AI20", "Mod2/AI21", "Mod2/AI22", "Mod2/AI23", "Mod2/AI24", "Mod2/AI25", "Mod2/AI26", "Mod2/AI27", "Mod2/AI28", "Mod2/AI29", "Mod2/AI30", "Mod2/AI31", "Mod3/AI0", "Mod3/AI1", "Mod3/AI2", "Mod3/AI3", "Mod3/AI4", "Mod3/AI5", "Mod3/AI6", "Mod3/AI7", "Mod3/AI8", "Mod3/AI9", "Mod3/AI10", "Mod3/AI11", "Mod3/AI12", "Mod3/AI13", "Mod3/AI14", "Mod3/AI15", "Mod3/AI16", "Mod3/AI17", "Mod3/AI18", "Mod3/AI19", "Mod3/AI20", "Mod3/AI21", "Mod3/AI22", "Mod3/AI23", "Mod3/AI24", "Mod3/AI25", "Mod3/AI26", "Mod3/AI27", "Mod3/AI28", "Mod3/AI29", "Mod3/AI30", "Mod3/AI31"] ("Array 2")
            n57 = Array Subset(array=w186, index=32 ("Index"), length=w185) -> (w182:string[])
            n58 = Array Subset(array=w186, index=0 ("Index"), length=w185) -> (w183:string[])
            n59 = Array Subset(array=w186, index=64 ("Index"), length=w185) -> (w181:string[])
            n60 = local write "Modul2/AIsNamen"(w182) -> ()
            n61 = local write "Modul1/AIsNamen"(w183) -> ()
            n62 = local write "Modul3/AIsNamen"(w181) -> ()
          }
        }
        n63 = Array Size(array="ReglerNameMod0") -> (size(s)=w169:i32)
        n64 = Array Size(array="ReglerNameMod1") -> (size(s)=w168:i32)
        n65 = Array Size(array="ReglerNameMod2A") -> (size(s)=w167:i32)
        n66 = Array Size(array="ReglerNameMod2B") -> (size(s)=w166:i32)
        n67 = Build Array "Anzahl Horst/Modul"(w169, w168, w167, w166) -> (w118:i32[])
        n68 = flat-sequence {
          tunnel: w118 -> [w179]
          tunnel: [w180] -> w117
          frame #0 {
            "AnzahlRegler/Modul" <- w179
          }
          frame #1 {
            n69 = local read "AnzahlRegler/Modul"() -> (w180:i32[])
          }
        }
        n70 = Build Array (concatenate)("Modul1/AIsNamen", "Modul2/AIsNamen", "Modul3/AIsNamen") -> (w119:string[])
        n71 = Bundle("DIOsMod0Nr"="DIOsMod0Nr", "DIOsMod1Nr"="DIOsMod1Nr", "DIOsMod2ANr"="DIOsMod2ANr", "DIOsMod2BNr"="DIOsMod2BNr", "AIsLH"="AIsLH", "AnzahlRegler/Modul"=w117, "Regler für den Probenfluß"="Regler für den Probenfluß", "SPvorgebenMod0"="SPvorgebenMod0", "SPvorgebenMod1"="SPvorgebenMod1", "SPvorgebenMod2A"="SPvorgebenMod2A", "SPvorgebenMod2B"="SPvorgebenMod2B", "MWAntwortMod0"="MWAntwortMod0", "MWAntwortMod1"="MWAntwortMod1", "MWAntwortMod2A"="MWAntwortMod2A", "MWAntwortMod2B"="MWAntwortMod2B", "FaktorMod0"="FaktorMod0", "FaktorMod1"="FaktorMod1", "FaktorMod2A"="FaktorMod2A", "FaktorMod2B"="FaktorMod2B", "MWabfragenMod0"="MWabfragenMod0", "MWabfragenMod1"="MWabfragenMod1", "MWabfragenMod2A"="MWabfragenMod2A", "MWabfragenMod2B"="MWabfragenMod2B", "Modul1/AI koeff"="Modul1/AI koeff", "Modul2/AI koeff"="Modul2/AI koeff", "Modul3/AI koeff"="Modul3/AI koeff", "Traps/MachsKoeff"="Traps/MachsKoeff", "Modul1/AIsNamen"="Modul1/AIsNamen", "Modul2/AIsNamen"="Modul2/AIsNamen", "Modul3/AIsNamen"="Modul3/AIsNamen", "DIOsMod0Name"="DIOsMod0Name", "DIOsMod1Name"="DIOsMod1Name", "DIOsMod2AName"="DIOsMod2AName", "DIOsMod2BName"="DIOsMod2BName", "ReglerNameMod0"="ReglerNameMod0", "ReglerNameMod1"="ReglerNameMod1", "ReglerNameMod2A"="ReglerNameMod2A", "ReglerNameMod2B"="ReglerNameMod2B", "Startmethode"="Startmethode", "Dateiordner Housekeeping"="Dateiordner Housekeeping", "Dateiname Housekeeping"="Dateiname Housekeeping", "DateiordnerECD1"="DateiordnerECD1", "DateinameECD1"="DateinameECD1", "DateiordnerECD2"="DateiordnerECD2", "DateinameECD2"="DateinameECD2", "NamenLangsameHeizungen"="NamenLangsameHeizungen", "ModuleLH"="ModuleLH", "Metavariablen"="Metavariablen") -> (w113:T4)  [unwired: 1 in]
        n72 = case shown="True" "EinstellungenSpeichern" {
          tunnel: w114 -> [_ w175]
          tunnel: w113 -> [_ w174]
          frame False {
          }
          frame True {
            n73 = Open/Create/Replace File(file path (use dialog)=w175, operation (0:open)=T5."replace" ("Operation (0:Öffnen)")) -> (refnum out=w177:refnum<file>, error out=w173:errorcluster)  [unwired: 4 in, 1 out]
            n74 = Write to Binary File(file (use dialog)=w177, data=w174, error in=w173) -> (refnum out=w176:refnum<file>, error out=w172:errorcluster)  [unwired: 3 in, 1 out]
            n75 = Close File(refnum=w176, error in=w172) -> (error out=w171:errorcluster)  [unwired: 1 out]
            n76 = call <vilib>:"Simple Error Handler.vi"("error in (no error)"=w171) -> ()  [unwired: 4 in, 5 out]
          }
        }
      }
      n77 = Build Array (concatenate)(w98, w99, w100, w101) -> (w97:string[])
    }
    frame #2 {
      w200 = string[] ["<", "<=", "=", ">=", ">", "=/="] ("Strings []")
      n78 = for {
        tunnel: w194 -> [w222] mode=indexing
        tunnel: [w220] -> w193 mode=indexing
        n79 = Concatenate Strings(w222, " heizen?" ("String")) -> (w220:string)
      }
      n80 = Build Array (concatenate)(w209, w208, w207, w206) -> (w204:string[])
      n81 = Build Array (concatenate)(w204, string[] ["Servo1 an", "Servo2 an", "Servo1 kalt", "Servo2 kalt", "Heizen?Trap1", "Heizen?Trap2", "Heizen?PreMach1", "Heizen?PreMach2", "Heizen?MainMach1", "Heizen?MainMach2", "Methodennummer", "STOPP!!!"], w193, w195, "PositionMPV", w190) -> (w202:string[])
      n82 = Build Array (concatenate)(w211, string[] ["T-Trap1", "T-Trap2", "T-PreMach1", "T-PreMach2", "T-MainMach1", "T-MainMach2"], w195, string[] ["Gesamte Zeit", "Methodenzeit", "Zykluszeit Mod0", "Zykluszeit Mod1", "Zykluszeit Mod2A", "Zykluszeit Mod2B"] ("Array"), "PositionMPV", w192) -> (w201:string[])
      n83 = property on="Vergleichsoperator2" class="Ring (strict)"("Strings []"=w200) -> ()  [unwired: 2 in, 2 out]
      n84 = while {
        tunnel: w219 -> [w291]
        tunnel: w218 -> [w290]
        tunnel: w217 -> [w289]
        tunnel: w216 -> [w288]
        tunnel: w215 -> [w287]
        tunnel: w214 -> [w286]
        tunnel: w213 -> [w285]
        tunnel: w212 -> [w284]
        shift-right: [w243] -> w196
        shift-left: w205 -> [w225]
        tunnel: w201 -> [w250]
        tunnel: w200 -> [w249]
        tunnel: w202 -> [w248]
        tunnel: w198 -> [w242]
        stop <- w281 stop-if-true
        n85 = Index Array(array=w225, index="Methode Nummer") -> (element=w280:T6)
        n86 = Unbundle(w280) -> ("Zykluslängen [s]"=w279:dbl[], "ZeitpktDIOsMod0"=w278:dbl[], "ZeitpktDIOsMod1"=w277:dbl[], "ZeitpktDIOsMod2A"=w276:dbl[], "ZeitpktDIOsMod2B"=w275:dbl[], "DIOsSPMod0"=w274:bool[][], "DIOsSPMod1"=w273:bool[][], "DIOsSPMod2A"=w272:bool[][], "DIOsSPMod2B"=w271:bool[][], "Mod0HorstZeitpkt"=w270:dbl[], "Mod1HorstZeitpkt"=w269:dbl[], "Mod2AHorstZeitpkt"=w268:dbl[], "Mod2BHorstZeitpkt"=w267:dbl[], "HorstSPMod0"=w266:dbl[][], "HorstSPMod1"=w265:dbl[][], "HorstSPMod2A"=w264:dbl[][], "HorstSPMod2B"=w263:dbl[][], "LHSetpoints"=w262:dbl[], "LHHeizen?"=w261:bool[], "ZPktFPGABoolesch"=w260:dbl[], "FPGABoolesch"=w259:bool[][], "ZeitpktFPGAPID"=w258:dbl[], "FPGAPID"=w257:T3, "ZeitpktFPGAFixp"=w256:dbl[], "SHSetpoints"=w255:dbl[][], "t_PreMach1"=w254:dbl[], "T_PreMach1"=w253:dbl[], "t_PreMach2"=w252:dbl[], "T_PreMach2"=w251:dbl[], "PIDs für \"träge\" Heizungen"=w247:T2, "Zwangsbedingungen"=w246:dbl[][], "Dateien fürs MS schicken?"=w245:bool, "ZeitpunkteMPV"=w238:dbl[], "SPMPV"=w237:i32[], "ZeitpktMS-1"=w240:dbl, "ZeitpktMS-2"=w239:dbl, "Int.Start1"=w236:dbl, "Int.Stop1"=w235:dbl, "Int.Start2"=w234:dbl, "Int.Stop2"=w233:dbl, "Methodenname"=w241:string, "t_MainMach1"=w232:dbl[], "T_MainMach1"=w231:dbl[], "t_MainMach2"=w230:dbl[], "T_MainMach2"=w229:dbl[])
        n87 = property on="LHHeizen?" class="Arr (strict)"("Value"=w261) -> ()  [unwired: 2 in, 2 out]
        n88 = property on="FPGAPID" class="Arr (strict)"("Value"=w257) -> ()  [unwired: 2 in, 2 out]
        n89 = property on="SPMPV" class="Arr (strict)"("Value"=w237) -> ()  [unwired: 2 in, 2 out]
        n90 = property on="Int.Start1" class="DigNum (strict)"("Value"=w236) -> ()  [unwired: 2 in, 2 out]
        n91 = property on="Int.Stop1" class="DigNum (strict)"("Value"=w235) -> ()  [unwired: 2 in, 2 out]
        n92 = property on="Int.Start2" class="DigNum (strict)"("Value"=w234) -> ()  [unwired: 2 in, 2 out]
        n93 = property on="Int.Stop2" class="DigNum (strict)"("Value"=w233) -> ()  [unwired: 2 in, 2 out]
        n94 = property on="T_MainMach2" class="Arr (strict)"("Value"=w229) -> ()  [unwired: 2 in, 2 out]
        n95 = property on="Zykluslängen [s]" class="Arr (strict)"("Value"=w279) -> ()  [unwired: 2 in, 2 out]
        n96 = property on="ZeitpktDIOsMod0" class="Arr (strict)"("Value"=w278) -> ()  [unwired: 2 in, 2 out]
        n97 = property on="Mod2BHorstZeitpkt" class="Arr (strict)"("Value"=w267) -> ()  [unwired: 2 in, 2 out]
        n98 = property on="HorstSPMod0" class="Arr (strict)"("Value"=w266) -> ()  [unwired: 2 in, 2 out]
        n99 = property on="LHSetpoints" class="Arr (strict)"("Value"=w262) -> ()  [unwired: 2 in, 2 out]
        n100 = property on="ZPktFPGABoolesch" class="Arr (strict)"("Value"=w260) -> ()  [unwired: 2 in, 2 out]
        n101 = property on="FPGABoolesch" class="Arr (strict)"("Value"=w259) -> ()  [unwired: 2 in, 2 out]
        n102 = property on="T_PreMach2" class="Arr (strict)"("Value"=w251) -> ()  [unwired: 2 in, 2 out]
        n103 = property on="PIDs für \"träge\" Heizungen" class="Arr (strict)"("Value"=w247) -> ()  [unwired: 2 in, 2 out]
        n104 = property on="DIOsSPMod1" class="Arr (strict)"("Value"=w273) -> ()  [unwired: 2 in, 2 out]
        n105 = property on="DIOsSPMod2A" class="Arr (strict)"("Value"=w272) -> ()  [unwired: 2 in, 2 out]
        n106 = property on="HorstSPMod1" class="Arr (strict)"("Value"=w265) -> ()  [unwired: 2 in, 2 out]
        n107 = property on="HorstSPMod2A" class="Arr (strict)"("Value"=w264) -> ()  [unwired: 2 in, 2 out]
        n108 = property on="HorstSPMod2B" class="Arr (strict)"("Value"=w263) -> ()  [unwired: 2 in, 2 out]
        n109 = property on="ZeitpktFPGAPID" class="Arr (strict)"("Value"=w258) -> ()  [unwired: 2 in, 2 out]
        n110 = property on="ZeitpktFPGAFixp" class="Arr (strict)"("Value"=w256) -> ()  [unwired: 2 in, 2 out]
        n111 = property on="SHSetpoints" class="Arr (strict)"("Value"=w255) -> ()  [unwired: 2 in, 2 out]
        n112 = property on="t_PreMach1" class="Arr (strict)"("Value"=w254) -> ()  [unwired: 2 in, 2 out]
        n113 = property on="T_PreMach1" class="Arr (strict)"("Value"=w253) -> ()  [unwired: 2 in, 2 out]
        n114 = property on="t_PreMach2" class="Arr (strict)"("Value"=w252) -> ()  [unwired: 2 in, 2 out]
        n115 = property on="ZeitpktDIOsMod1" class="Arr (strict)"("Value"=w277) -> ()  [unwired: 2 in, 2 out]
        n116 = property on="ZeitpktDIOsMod2A" class="Arr (strict)"("Value"=w276) -> ()  [unwired: 2 in, 2 out]
        n117 = property on="ZeitpktDIOsMod2B" class="Arr (strict)"("Value"=w275) -> ()  [unwired: 2 in, 2 out]
        n118 = property on="DIOsSPMod0" class="Arr (strict)"("Value"=w274) -> ()  [unwired: 2 in, 2 out]
        n119 = property on="DIOsSPMod2B" class="Arr (strict)"("Value"=w271) -> ()  [unwired: 2 in, 2 out]
        n120 = property on="Mod0HorstZeitpkt" class="Arr (strict)"("Value"=w270) -> ()  [unwired: 2 in, 2 out]
        n121 = property on="Mod1HorstZeitpkt" class="Arr (strict)"("Value"=w269) -> ()  [unwired: 2 in, 2 out]
        n122 = property on="Mod2AHorstZeitpkt" class="Arr (strict)"("Value"=w268) -> ()  [unwired: 2 in, 2 out]
        n123 = property on="Dateien fürs MS schicken?" class="Bool (strict)"("Value"=w245) -> ()  [unwired: 2 in, 2 out]
        n124 = property on="ZeitpunkteMPV" class="Arr (strict)"("Value"=w238) -> ()  [unwired: 2 in, 2 out]
        n125 = property on="ZeitpktMS-1" class="DigNum (strict)"("Value"=w240) -> ()  [unwired: 2 in, 2 out]
        n126 = property on="ZeitpktMS-2" class="DigNum (strict)"("Value"=w239) -> ()  [unwired: 2 in, 2 out]
        n127 = property on="Methodenname" class="Str"("Value"=w241) -> ()  [unwired: 2 in, 2 out]
        n128 = property on="t_MainMach1" class="Arr (strict)"("Value"=w232) -> ()  [unwired: 2 in, 2 out]
        n129 = property on="T_MainMach1" class="Arr (strict)"("Value"=w231) -> ()  [unwired: 2 in, 2 out]
        n130 = property on="t_MainMach2" class="Arr (strict)"("Value"=w230) -> ()  [unwired: 2 in, 2 out]
        n131 = while {
          tunnel: w290 -> [w399]
          tunnel: w289 -> [w398]
          tunnel: w288 -> [w397]
          tunnel: w287 -> [w396]
          tunnel: w286 -> [w395]
          tunnel: w284 -> [w394]
          tunnel: w285 -> [w393]
          tunnel: w291 -> [w363]
          tunnel: [w362] -> w282
          tunnel: [w325] -> w283
          tunnel: ["EditorBeenden"] -> w281
          tunnel: w250 -> [w348]
          shift-right: [w343] -> _
          shift-left: w246 -> [w347]
          tunnel: w249 -> [w346]
          tunnel: w248 -> [w345]
          tunnel: ["AllesSpeichern"] -> w244
          tunnel: ["MethodeDuplizieren"] -> w227
          stop <- w317 stop-if-true
          n132 = for {
            tunnel: w347 -> [w408] mode=indexing
            tunnel: w348 -> [w404]
            tunnel: w346 -> [w403]
            tunnel: w345 -> [w422]
            tunnel: [w416] -> w356 mode=indexing
            n133 = Index Array(array=w408, index=0 ("Index")) -> (element=w428:dbl)
            n134 = Index Array(array=w408, index=1 ("Index")) -> (element=w426:dbl)
            n135 = Index Array(array=w408, index=3 ("Index")) -> (element=w410:dbl)
            n136 = Index Array(array=w408, index=4 ("Index")) -> (element=w409:dbl)
            n137 = Index Array(array=w408, index=6 ("Index")) -> (element=w424:dbl)
            n138 = To Long Integer(number=w428) -> (32bit integer=w427:i32)
            n139 = To Long Integer(number=w426) -> (32bit integer=w425:i32)
            n140 = To Long Integer(number=w410) -> (32bit integer=w407:i32)
            n141 = To Long Integer(number=w409) -> (32bit integer=w406:i32)
            n142 = To Long Integer(number=w424) -> (32bit integer=w423:i32)
            n143 = Index Array(array=w408, index=2 ("Index")) -> (element=w421:dbl)
            n144 = Index Array(array=w408, index=5 ("Index")) -> (element=w405:dbl)
            n145 = Index Array(array=w408, index=7 ("Index")) -> (element=w420:dbl)
            n146 = Index Array(array=w404, index=w427) -> (element=w419:string)
            n147 = Index Array(array=w403, index=w425) -> (element=w418:string)
            n148 = Index Array(array=w404, index=w407) -> (element=w402:string)
            n149 = Index Array(array=w403, index=w406) -> (element=w401:string)
            n150 = Index Array(array=w422, index=w423) -> (element=w414:string)
            n151 = Number To Exponential String(number=w421) -> (E-format string=w417:string)  [unwired: 3 in]
            n152 = Number To Exponential String(number=w405) -> (E-format string=w400:string)  [unwired: 3 in]
            n153 = Number To Exponential String(number=w420) -> (E-format string=w415:string)  [unwired: 3 in]
            n154 = Build Array(w419, w418, w417, w402, w401, w400, w414, w415) -> (w416:string[])
          }
          "ZwangsBedingungen" <- w356
          n155 = Wait (ms)(milliseconds to wait=u32 500 ("Zu wartende ms")) -> ()  [unwired: 1 out]
          n156 = Build Array("AbfragbareVariablen1", "Vergleichsoperator1", "Wert1", "AbfragbareVariablen2", "Vergleichsoperator2", "Wert2", "BedienbareVariablen", "Ausgangswert") -> (w353:dbl[])
          n157 = case shown="False" "Bedingung übernehmen" {
            tunnel: w347 -> [w438 w441]
            tunnel: w353 -> [_ w440]
            tunnel: [w438 w439] -> w354
            frame False {
            }
            frame True {
              n158 = Build Array (concatenate)(w441, w440) -> (w439:dbl[][])
            }
          }
          n159 = case shown="True" "löschen" {
            tunnel: w354 -> [w434 w437]
            tunnel: [w434 w435] -> w343
            frame False {
            }
            frame True {
              n160 = Delete From Array(array=w437, index (row)="Bedingung Nr. X") -> (array with subset deleted=w435:dbl[][])  [unwired: 2 in, 1 out]
            }
          }
          n161 = Or(x="MethodeSpeichern", y="EditorBeenden") -> (x .or. y?=w360:bool)
          n162 = Or(x=w360, y="MethodeLaden") -> (x .or. y?=w327:bool)
          n163 = local write "Zwangsbedingungen"(w343) -> ()
          n164 = Or(x=w327, y="AllesSpeichern") -> (x .or. y?=w318:bool)
          n165 = Or(x="MethodeDuplizieren", y=w318) -> (x .or. y?=w317:bool)
          n166 = Or(x="AllesSpeichern", y="MethodeSpeichern") -> (x .or. y?=w325:bool)
          n167 = Bundle("Zykluslängen [s]"="Zykluslängen [s]", "ZeitpktDIOsMod0"="ZeitpktDIOsMod0", "ZeitpktDIOsMod1"="ZeitpktDIOsMod1", "ZeitpktDIOsMod2A"="ZeitpktDIOsMod2A", "ZeitpktDIOsMod2B"="ZeitpktDIOsMod2B", "DIOsSPMod0"="DIOsSPMod0", "DIOsSPMod1"="DIOsSPMod1", "DIOsSPMod2A"="DIOsSPMod2A", "DIOsSPMod2B"="DIOsSPMod2B", "Mod0HorstZeitpkt"="Mod0HorstZeitpkt", "Mod1HorstZeitpkt"="Mod1HorstZeitpkt", "Mod2AHorstZeitpkt"="Mod2AHorstZeitpkt", "Mod2BHorstZeitpkt"="Mod2BHorstZeitpkt", "HorstSPMod0"="HorstSPMod0", "HorstSPMod1"="HorstSPMod1", "HorstSPMod2A"="HorstSPMod2A", "HorstSPMod2B"="HorstSPMod2B", "LHSetpoints"="LHSetpoints", "LHHeizen?"="LHHeizen?", "ZPktFPGABoolesch"="ZPktFPGABoolesch", "FPGABoolesch"="FPGABoolesch", "ZeitpktFPGAPID"="ZeitpktFPGAPID", "FPGAPID"="FPGAPID", "ZeitpktFPGAFixp"="ZeitpktFPGAFixp", "SHSetpoints"="SHSetpoints", "t_PreMach1"="t_PreMach1", "T_PreMach1"="T_PreMach1", "t_PreMach2"="t_PreMach2", "T_PreMach2"="T_PreMach2", "PIDs für \"träge\" Heizungen"="PIDs für \"träge\" Heizungen", "Zwangsbedingungen"="Zwangsbedingungen", "Dateien fürs MS schicken?"="Dateien fürs MS schicken?", "ZeitpunkteMPV"="ZeitpunkteMPV", "SPMPV"="SPMPV", "ZeitpktMS-1"="ZeitpktMS-1", "ZeitpktMS-2"="ZeitpktMS-2", "Int.Start1"="Int.Start1", "Int.Stop1"="Int.Stop1", "Int.Start2"="Int.Start2", "Int.Stop2"="Int.Stop2", "Methodenname"="Methodenname", "t_MainMach1"="t_MainMach1", "T_MainMach1"="T_MainMach1", "t_MainMach2"="t_MainMach2", "T_MainMach2"="T_MainMach2") -> (w362:T6)  [unwired: 1 in]
          "DIOsMod0Name" <- w363
          "DIOsMod1Name" <- w399
          "DIOsMod2AName" <- w398
          "DIOsMod2BName" <- w397
          "HorstMod0Name" <- w396
          "HorstMod2BName" <- w393
          "HorstMod2AName" <- w394
          "HorstMod1Name" <- w395
        }
        n168 = case shown="True" "MethodeLöschen" {
          tunnel: w225 -> [w292 w296]
          tunnel: [w292 w293] -> w224
          tunnel: "Methode Nummer" -> [_ w294]
          frame False {
          }
          frame True {
            n169 = invoke on="MethodeLöschen" class="Bool (strict)" method="Reinit To Default"() -> ()  [unwired: 3 in, 3 out]
            n170 = Delete From Array(array=w296, length=1, index=w294) -> (array with subset deleted=w293:T1)  [unwired: 1 out]
          }
        }
        n171 = case shown="True" w227 {
          tunnel: w224 -> [w297 w300]
          tunnel: [w297 w299] -> w228
          tunnel: "Methode Nummer" -> [_ w301]
          frame False {
          }
          frame True {
            n172 = Index Array(array=w300, index=w301) -> (element=w298:T6)
            n173 = Build Array (concatenate)(w300, w298) -> (w299:T1)
          }
        }
        n174 = case shown="True" w283 {
          tunnel: w228 -> [w310 w316]
          tunnel: w282 -> [_ w311]
          tunnel: [w310 w312] -> w243
          tunnel: "Methode Nummer" -> [_ w313]
          frame False {
          }
          frame True {
            n175 = Delete From Array(array=w316, length=1 ("Länge"), index=w313) -> (array with subset deleted=w314:T1)  [unwired: 1 out]
            n176 = Insert Into Array(array=w314, index=w313, new element=w311) -> (w312:T1)
          }
        }
        n177 = case shown="True" w244 {
          tunnel: w243 -> [_ w307]
          tunnel: w242 -> [_ w302]
          frame False {
          }
          frame True {
            n178 = Open/Create/Replace File(file path (use dialog)=w302, operation (0:open)=T5."replace" ("Operation (0:Öffnen)")) -> (refnum out=w306:refnum<file>, error out=w308:errorcluster)  [unwired: 4 in, 1 out]
            n179 = Write to Binary File(file (use dialog)=w306, data=w307, error in=w308) -> (refnum out=w304:refnum<file>, error out=w305:errorcluster)  [unwired: 3 in, 1 out]
            n180 = Close File(refnum=w304, error in=w305) -> (error out=w303:errorcluster)  [unwired: 1 out]
            n181 = call <vilib>:"Simple Error Handler.vi"("error in (no error)"=w303) -> ()  [unwired: 4 in, 5 out]
          }
        }
      }
      "Methoden" <- w196
      n182 = property on="BedienbareVariablen" class="Ring (strict)"("Strings []"=w202) -> ()  [unwired: 2 in, 2 out]
      n183 = property on="AbfragbareVariablen1" class="Ring (strict)"("Strings []"=w201) -> ()  [unwired: 2 in, 2 out]
      n184 = property on="AbfragbareVariablen2" class="Ring (strict)"("Strings []"=w201) -> ()  [unwired: 2 in, 2 out]
      n185 = property on="Vergleichsoperator1" class="Ring (strict)"("Strings []"=w200) -> ()  [unwired: 2 in, 2 out]
      "LangsameHeizungen" <- w199
    }
  }
  n186 = Close File(refnum=w19, error in=w18) -> (path=w16:path, error out=w17:errorcluster)
  n187 = call <vilib>:"Simple Error Handler.vi"("error in (no error)"=w17) -> ()  [unwired: 4 in, 5 out]
  n188 = Open/Create/Replace File(file path (use dialog)=path "C:/methoden.per" ("Dateipfad Methoden")) -> (refnum out=w14:refnum<file>, error out=w13:errorcluster)  [unwired: 5 in, 1 out]
  n189 = Read from Binary File(5:T1 [], 8:w13, 11:w14) -> (0:w11:errorcluster, 2:w6:T1, 3:w12:refnum<file>)  [unwired: 3 in, 1 out]
  n190 = Close File(refnum=w12, error in=w11) -> (path=w9:path, error out=w10:errorcluster)
  "error out" <- w10
  n191 = call <vilib>:"Simple Error Handler.vi"("error in (no error)"=w10) -> ()  [unwired: 4 in, 5 out]
